vi "Exp_Setup_Control_remote.vi"(2 "Dispersion?":bool) -> ()   [LabVIEW 2010]
uses:
  ADAM Controls/Remember_value_mode.ctl
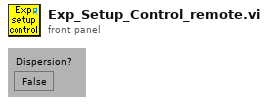
[diagram p1: front panel]
types:
  T1 = typedef "Remember_value_mode.ctl" = enum16{"Read only", "Read and Write"}
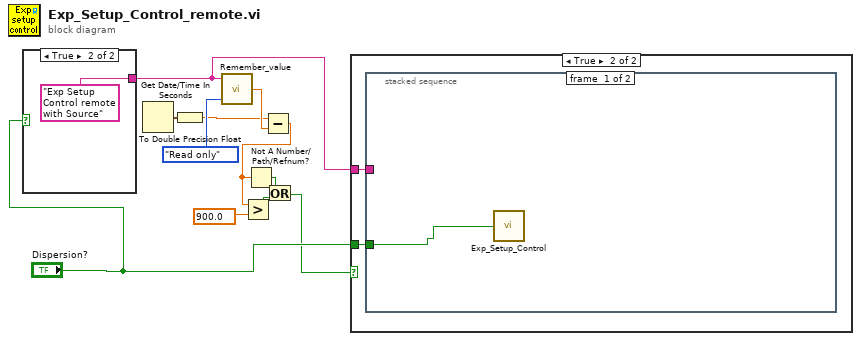
[diagram p0: block diagram]
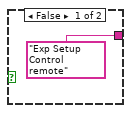
[diagram p2: hidden frame]
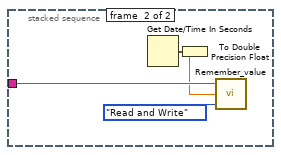
[diagram p4: hidden frame]
diagram:
  n1 = case shown="True" "Dispersion?" {
    tunnel: ["Exp Setup Control remote" ("Ch name") "Exp Setup Control remote with Source" ("Ch name")] -> w4
    frame False {
    }
    frame True {
    }
  }
  n2 = Get Date/Time In Seconds() -> (seconds since 1Jan1904=w1:timestamp)
  n3 = To Double Precision Float(number=w1) -> (double precision float=w5:dbl)
  n4 = call "Remember_value.vi"("Mode"=Remember_value_mode."Read only", "Ch name"=w4) -> ("Output Value"=w9:dbl)  [unwired: 1 in]
  n5 = Subtract(x=w5, y=w9) -> (x-y=w8:dbl)
  n6 = Greater?(x=w8, y=900.0) -> (0:w7:bool)
  n7 = Not A Number/Path/Refnum?(number/path/refnum=w8) -> (NaN/Path/Refnum?=w6:bool)
  n8 = Or(x=w6, y=w7) -> (x .or. y?=w2:bool)
  n9 = case shown="True" w2 {
    tunnel: "Dispersion?" -> [_ w15]
    tunnel: w4 -> [_ w14]
    frame False {
    }
    frame True {
      n10 = stacked-sequence {
        tunnel: w15 -> [w16 _]
        tunnel: w14 -> [_ w20]
        frame #0 {
          n11 = call "Exp_Setup_Control.vi"("Dispersion?"=w16) -> ()  [unwired: 3 out]
        }
        frame #1 {
          n12 = Get Date/Time In Seconds() -> (seconds since 1Jan1904=w17:timestamp)
          n13 = To Double Precision Float(number=w17) -> (double precision float=w18:dbl)
          n14 = call "Remember_value.vi"("Mode"=Remember_value_mode."Read and Write", "Input Value"=w18, "Ch name"=w20) -> ()  [unwired: 1 out]
        }
      }
    }
  }
